vi "prototipo.vi"() -> ()   [LabVIEW 2021]
uses:
  <vilib>/Instr/_visa.llb/VISA Configure Serial Port (Instr).vi
  <vilib>/addons/control/pid/pid.llb/PID (DBL).vi
  <vilib>/Utility/file.llb/Write Delimited Spreadsheet (DBL).vi
  <vilib>/addons/control/pid/NI_PID_pid.lvlib
panel:
  in  "stop 2":bool
  out "dt out (s)":dbl format="%.3f"
  out "Velocità 2":dbl(knob) scale=0.0..1300.0
  out "velocità 2":dbl
  in  "PWM.txt":path
  in  "data bits (8)":u16=8 min=5 max=8 step=1
  in  "baud rate (9600)":u32=9600
  in  "VISA resource name":refnum<visa-resource-name>
  out "Numero iterazioni":i32
  in  "setpoint":dbl format="%.2f"
  out "SP & PV":cluster{"initial PV":dbl, "SP:":dbl}(graph)
  in  "PID gains":T1={"proportional gain (Kc)"=1.0, "integral time (Ti, min)"=0.01, "derivative time (Td, min)"=0.0} {"derivative time (Td, min)" format="%.3f"; "integral time (Ti, min)" format="%.3f"; "proportional gain (Kc)" format="%.3f"}
  out "Thermometer":dbl(slide) scale=0.0..100.0
  in  "dt (s)":dbl=-1.0 format="%.3f"
  in  "output range":cluster{"output high":dbl, "output low":dbl}={"output high"=100.0, "output low"=-100.0} {"output low" format="%.2f"; "output high" format="%.2f"}
  out "PWM":dbl format="%.2f"
  out "MV":dbl(graph)
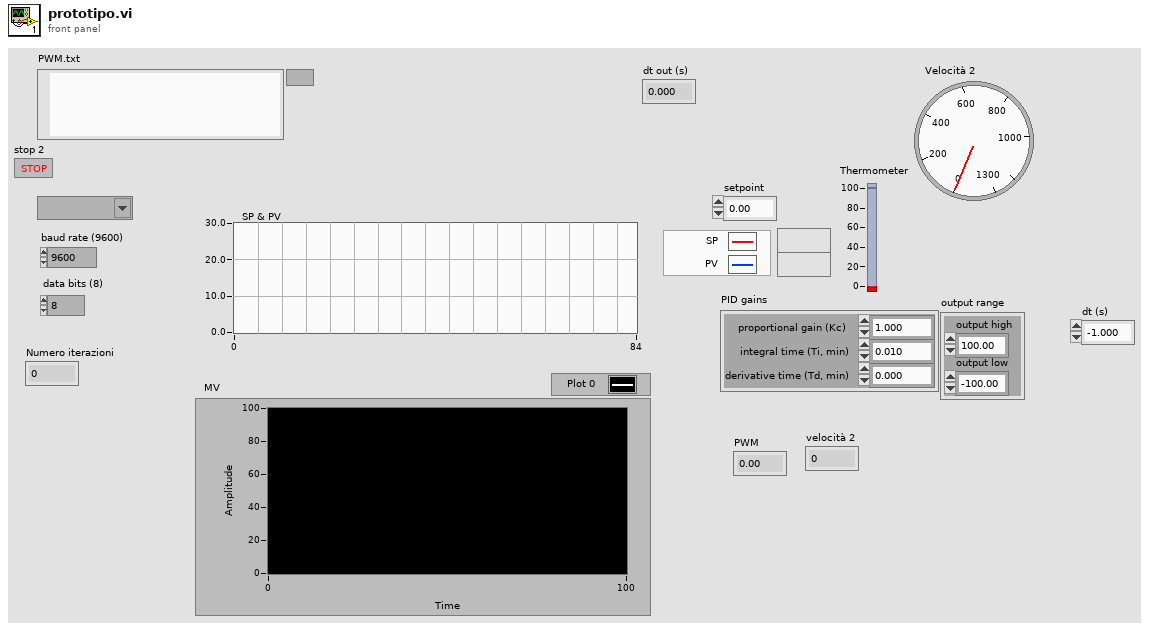
[diagram p1: front panel]
types:
  T1 = cluster{"proportional gain (Kc)":dbl, "integral time (Ti, min)":dbl, "derivative time (Td, min)":dbl}
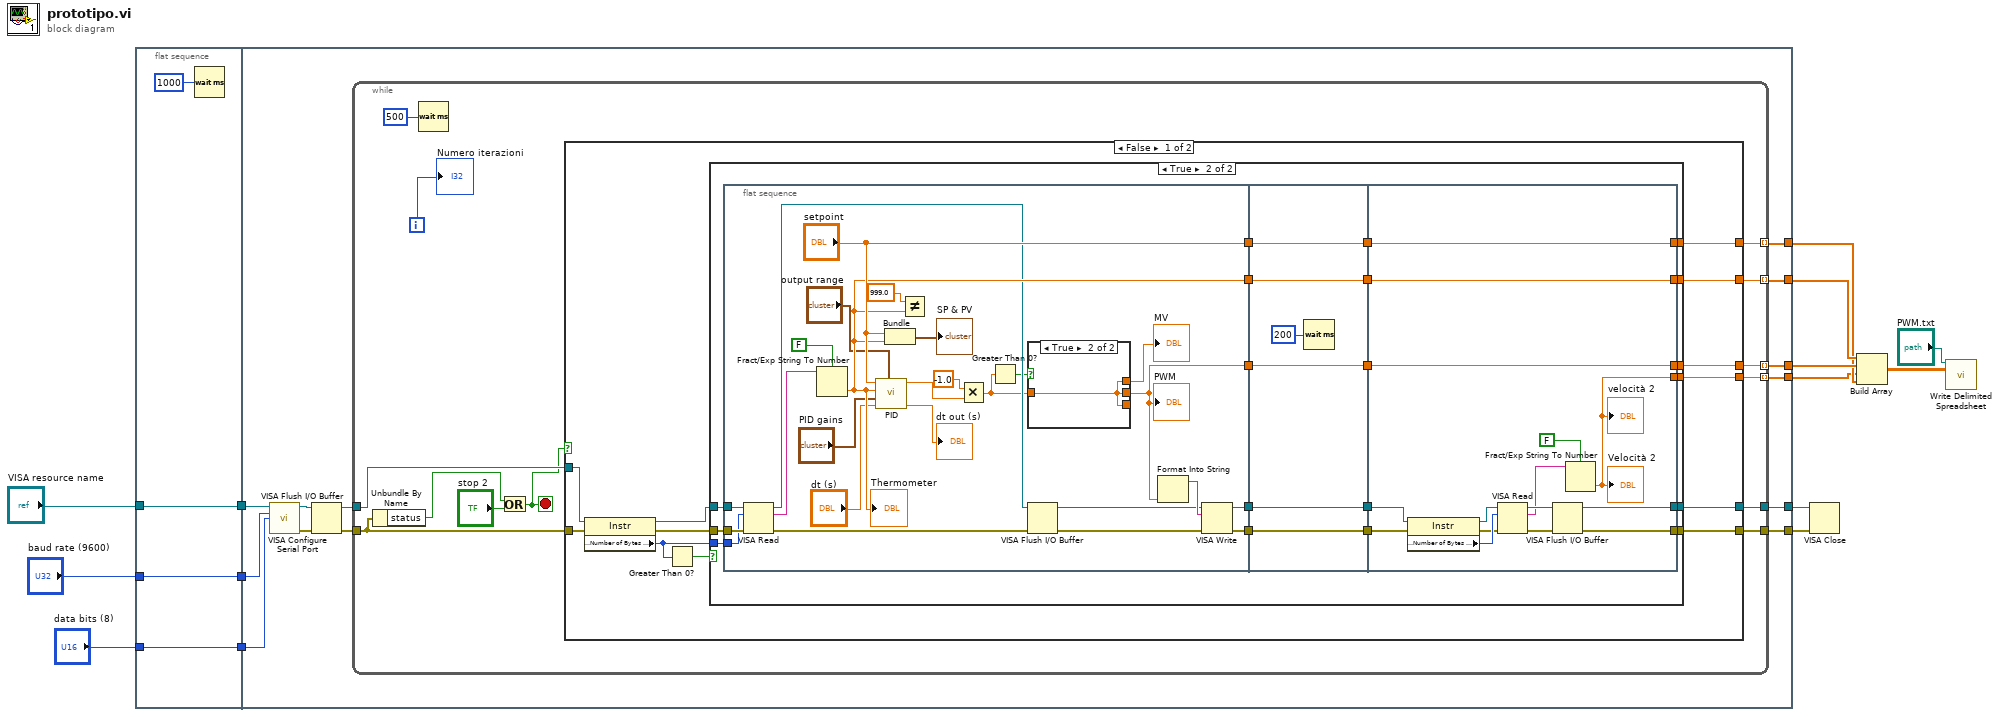
[diagram p0: block diagram]
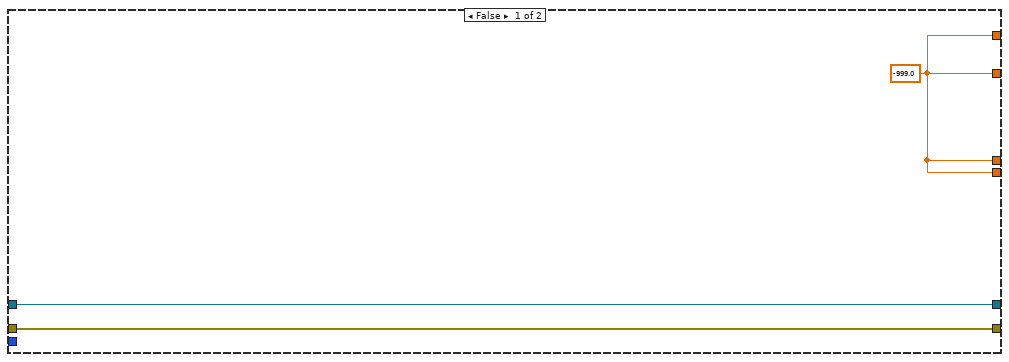
[diagram p2: hidden frame]
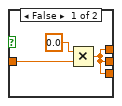
[diagram p3: hidden frame]
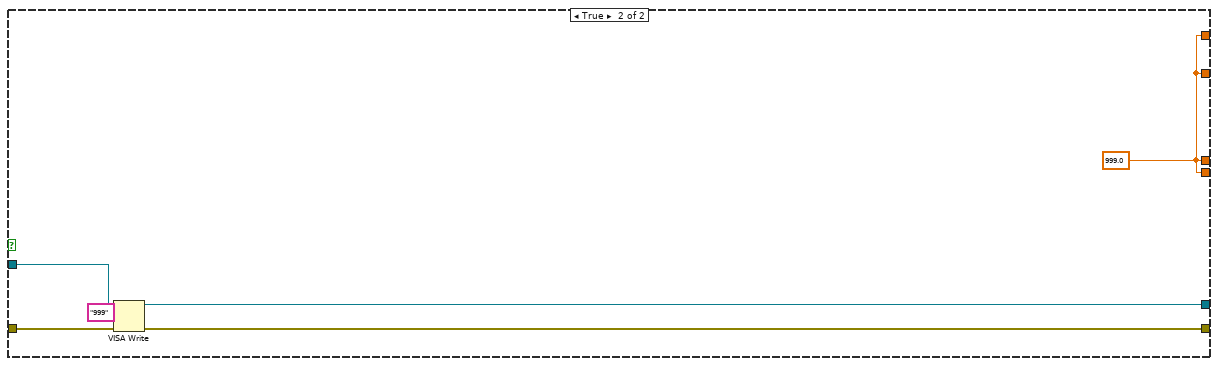
[diagram p4: hidden frame]
diagram:
  n1 = flat-sequence {
    tunnel: "baud rate (9600)" -> [w16]
    tunnel: "data bits (8)" -> [w17]
    tunnel: "VISA resource name" -> [w18]
    tunnel: [w18] -> w5
    tunnel: [w17] -> w4
    tunnel: [w16] -> w3
    tunnel: [w28] -> w10
    tunnel: [w27] -> w9
    tunnel: [w26] -> w7
    tunnel: [w25] -> w6
    tunnel: w5 -> [w29]
    tunnel: w4 -> [w30]
    tunnel: w3 -> [w31]
    tunnel: [w20] -> w2
    tunnel: [w19] -> w1
    frame #0 {
      n2 = Wait (ms)(milliseconds to wait=u32 1000) -> ()  [unwired: 1 out]
    }
    frame #1 {
      n3 = call-poly "VISA Configure Serial Port"("VISA resource name"=w29, "baud rate (9600)"=w31, "data bits (8)"=w30) -> ("VISA resource name out"=w21:refnum<visa-resource-name>, "error out"=w24:errorcluster)  [unwired: 11 in]
      n4 = VISA Flush I/O Buffer(VISA resource name=w21, error in (no error)=w24) -> (VISA resource name out=w23:refnum<visa-resource-name>, error out=w22:errorcluster)  [unwired: 1 in]
      n5 = while {
        tunnel: [w43] -> w27 mode=indexing
        tunnel: [w42] -> w28
        tunnel: [w41] -> w26 mode=indexing
        tunnel: [w40] -> w25 mode=indexing
        tunnel: w23 -> [w39]
        tunnel: w22 -> [w35]
        tunnel: [w38] -> w20 mode=indexing
        tunnel: [w37] -> w19
        i -> [w44]
        stop <- w32 stop-if-true
        n6 = Unbundle By Name(w35) -> ("status"=w33:bool)
        n7 = Wait (ms)(milliseconds to wait=u32 500) -> ()  [unwired: 1 out]
        n8 = Or(x=w33, y="stop 2") -> (x .or. y?=w32:bool)
        n9 = case shown="False" w32 {
          tunnel: [w56 w135] -> w43
          tunnel: [w55 w130] -> w42
          tunnel: [w54 w135] -> w41
          tunnel: [w53 w135] -> w40
          tunnel: w39 -> [w52 w133]
          tunnel: w35 -> [w51 w132]
          tunnel: [w50 w135] -> w38
          tunnel: [w49 w131] -> w37
          frame False {
            n10 = property class="Instr"(reference=w52, error in=w51) -> (reference out=w48:refnum<visa-resource-name>, error out=w47:errorcluster, "Serial Settings:Number of Bytes at Serial Port"=w45:u32)
            n11 = Greater Than 0?(x=w45) -> (x > 0?=w46:bool)
            n12 = case shown="True" w46 {
              tunnel: [w57 w71] -> w56
              tunnel: [w58 w78] -> w55
              tunnel: [w57 w77] -> w54
              tunnel: [w57 w76] -> w53
              tunnel: [w57 w75] -> w50
              tunnel: [w59 w74] -> w49
              tunnel: w48 -> [w59 w73]
              tunnel: w47 -> [w58 w72]
              tunnel: w45 -> [_ w70]
              frame False {
                w57 = -999.0
              }
              frame True {
                n13 = flat-sequence {
                  tunnel: w73 -> [w102]
                  tunnel: w72 -> [w101]
                  tunnel: w70 -> [w91]
                  tunnel: [w104] -> w69
                  tunnel: ["setpoint"] -> w67
                  tunnel: [w98] -> w65
                  tunnel: [w80] -> w63
                  tunnel: [w79] -> w61
                  tunnel: w69 -> [w114]
                  tunnel: [w114] -> w68
                  tunnel: w67 -> [w113]
                  tunnel: [w113] -> w66
                  tunnel: w65 -> [w112]
                  tunnel: [w112] -> w64
                  tunnel: w63 -> [w111]
                  tunnel: [w111] -> w62
                  tunnel: w61 -> [w110]
                  tunnel: [w110] -> w60
                  tunnel: [w127] -> w71
                  tunnel: [w115] -> w74
                  tunnel: [w117] -> w75
                  tunnel: [w128] -> w76
                  tunnel: [w129] -> w77
                  tunnel: [w116] -> w78
                  tunnel: w68 -> [w129]
                  tunnel: w66 -> [w128]
                  tunnel: w64 -> [w127]
                  tunnel: w62 -> [w119]
                  tunnel: w60 -> [w118]
                  frame #0 {
                    n14 = VISA Read(VISA resource name=w102, byte count=w91, error in (no error)=w101) -> (VISA resource name out=w93:refnum<visa-resource-name>, read buffer=w100:string, error out=w94:errorcluster)  [unwired: 1 out]
                    n15 = Fract/Exp String To Number(use system decimal point (T)=FALSE, string=w100) -> (number=w98:dbl)  [unwired: 2 in, 1 out]
                    "Thermometer" <- w98
                    n16 = call-poly <vilib>:"PID.vi"("output range"="output range", "dt (s)"="dt (s)", "PID gains"="PID gains", "process variable"=w98, "setpoint"="setpoint") -> ("dt out (s)"=→"dt out (s)":dbl, "output"=w83:dbl)  [unwired: 5 in]
                    n17 = Bundle("setpoint"="setpoint", w98) -> (→"SP & PV":cluster{"setpoint":dbl, dbl})  [unwired: 1 in]
                    n18 = Not Equal?(x=999.0, y=w98) -> ()  [unwired: 1 out]
                    n19 = Multiply(x=-1.0, y=w83) -> (x*y=w81:dbl)
                    n20 = Greater Than 0?(x=w81) -> (x > 0?=w84:bool)
                    n21 = case shown="True" w84 {
                      tunnel: [w106 w108] -> w104
                      tunnel: [w106 w108] -> _
                      tunnel: [w106 w108] -> w90
                      tunnel: w81 -> [w105 w108]
                      frame False {
                        n22 = Multiply(x=0.0, y=w105) -> (x*y=w106:dbl)
                      }
                      frame True {
                      }
                    }
                    "PWM" <- w104
                    "MV" <- w90
                    n23 = VISA Flush I/O Buffer(VISA resource name=w93, error in (no error)=w94) -> (VISA resource name out=w96:refnum<visa-resource-name>, error out=w95:errorcluster)  [unwired: 1 in]
                    n24 = Format Into String(w104) -> (resulting string=w97:string)  [unwired: 3 in, 1 out]
                    n25 = VISA Write(VISA resource name=w96, write buffer=w97, error in (no error)=w95) -> (VISA resource name out=w80:refnum<visa-resource-name>, error out=w79:errorcluster)  [unwired: 1 out]
                  }
                  frame #1 {
                    n26 = Wait (ms)(milliseconds to wait=u32 200) -> ()  [unwired: 1 out]
                  }
                  frame #2 {
                    n27 = property class="Instr"(reference=w119, error in=w118) -> (reference out=w121:refnum<visa-resource-name>, error out=w122:errorcluster, "Serial Settings:Number of Bytes at Serial Port"=w123:u32)
                    n28 = VISA Read(VISA resource name=w121, byte count=w123, error in (no error)=w122) -> (VISA resource name out=w126:refnum<visa-resource-name>, read buffer=w124:string, error out=w125:errorcluster)  [unwired: 1 out]
                    n29 = VISA Flush I/O Buffer(VISA resource name=w126, error in (no error)=w125) -> (VISA resource name out=w115:refnum<visa-resource-name>, error out=w116:errorcluster)  [unwired: 1 in]
                    n30 = Fract/Exp String To Number(use system decimal point (T)=FALSE, string=w124) -> (number=w117:dbl)  [unwired: 2 in, 1 out]
                    "velocità 2" <- w117
                    "Velocità 2" <- w117
                  }
                }
              }
            }
          }
          frame True {
            w135 = 999.0
            n31 = VISA Write(VISA resource name=w133, write buffer="999", error in (no error)=w132) -> (VISA resource name out=w131:refnum<visa-resource-name>, error out=w130:errorcluster)  [unwired: 1 out]
          }
        }
        "Numero iterazioni" <- w44
      }
    }
  }
  n32 = VISA Close(VISA resource name=w1, error in (no error)=w10) -> ()  [unwired: 1 out]
  n33 = Build Array(w9, w7, w2, w6) -> (w8:dbl[][])
  n34 = call-poly <vilib>:"Write Delimited Spreadsheet.vi"("file path (dialog if empty)"="PWM.txt", "2D data"=w8) -> ()  [unwired: 12 in, 2 out]
